vi "PerformanceAnalizer.vi"() -> ()   [LabVIEW 2010]
uses:
  <vilib>/picture/picture.llb/Draw True-Color Pixmap.vi
  <vilib>/Utility/file.llb/Write To Spreadsheet File (DBL).vi
  <vilib>/Utility/file.llb/Write To Spreadsheet File (string).vi
panel:
  out "KTH  Automatic Control \nCommunication performance analyzer":picture
  in  "Tab Control":T1(tab)
  out "reliability =pckSuccess/pckTotal":dynamicdata(graph)
  out "errors":dynamicdata(graph)
  out "Inter sampling time = t_k - t_k-1":dynamicdata(graph)
  out "delay = t_send - t_ack":dynamicdata(graph)
  out "lqi":dynamicdata(graph)
  out "rssi":dynamicdata(graph)
  out "rssi_0":i8
  out "rssi_1":i8
  out "rssi_2":i8
  out "lqi_0":i8
  out "lqi_1":i8
  out "lqi_2":i8
  in  "StartSaving":bool
  in  "Saving":bool
  in  "StopSaving":bool
  out "Path":path
  out "errors_0":dbl
  out "errors_2":dbl
  out "delay_1":dbl
  out "delay_0":dbl
  out "delay_2":dbl
  out "interSampling_1":dbl
  out "interSampling_3":dbl
  out "interSampling_0":dbl
  out "errors_1":dbl
  out "reliability_0":dbl
  out "reliability_1":dbl
  out "reliability_2":dbl
  out "current time":timestamp
  out "Packet Window":i32=200
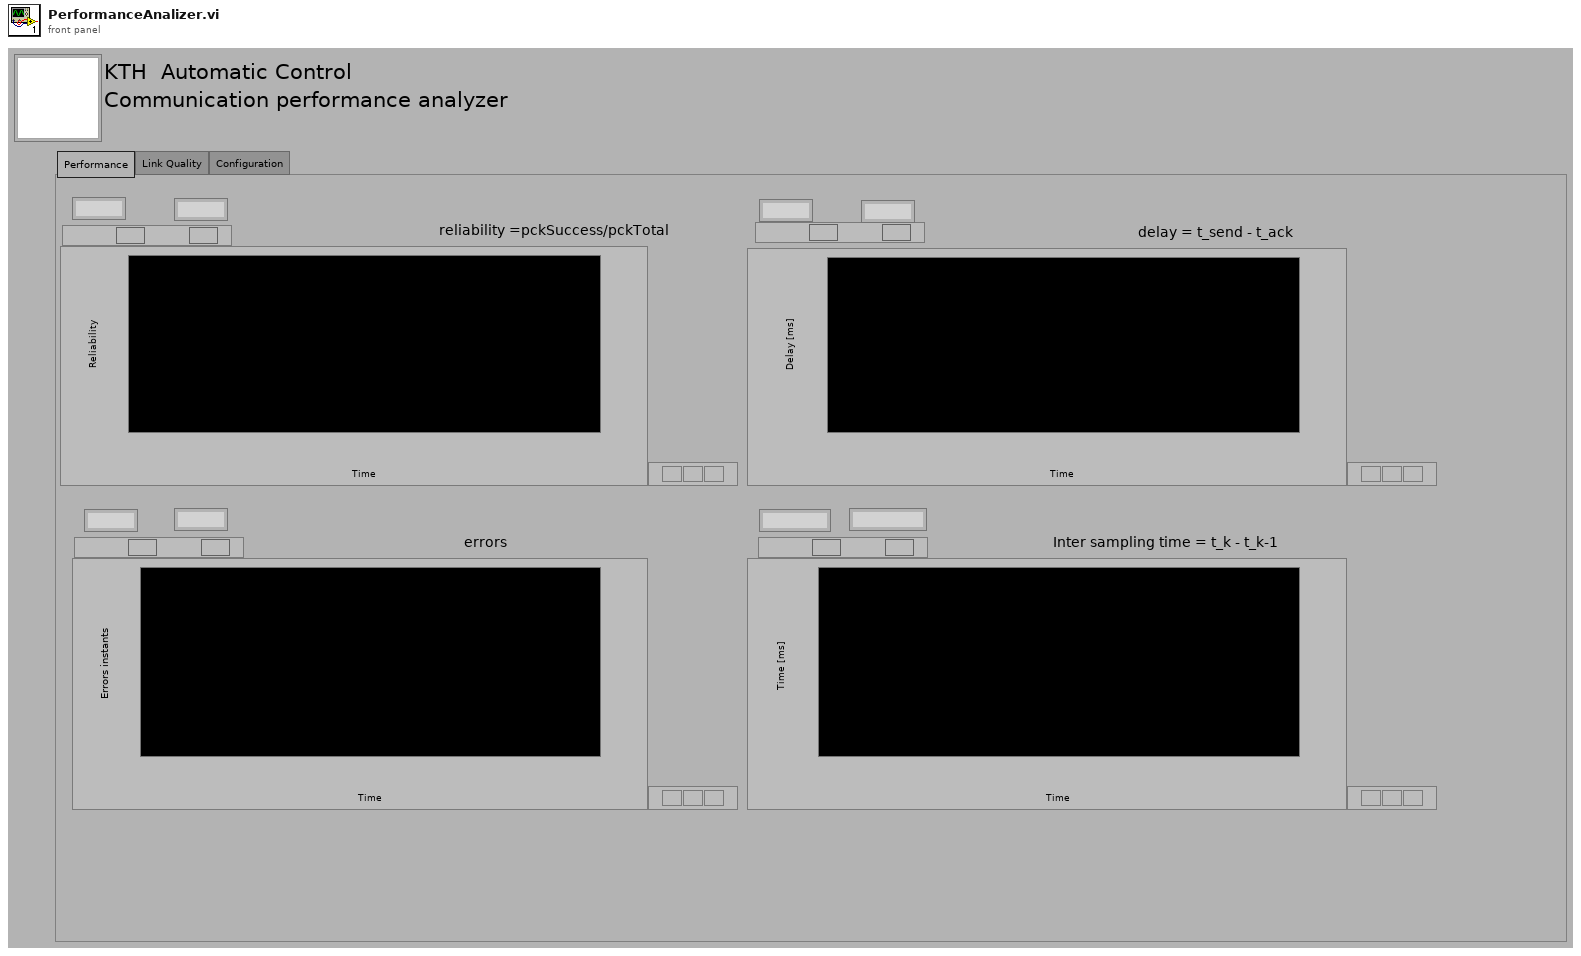
[diagram p1: front panel]
types:
  T1 = enum32{"Performance", "Link Quality", "Configuration"}
  T2 = enum8{"Enabled", "Disabled", "Disabled and Grayed Out"}
  T3 = typedef "imagedata.ctl" = cluster{"image type":i32, "image depth":i32, "image":u8[], "mask":u8[], "colors":u32[], "Rectangle":cluster{"left":i16, "top":i16, "right":i16, "bottom":i16}}
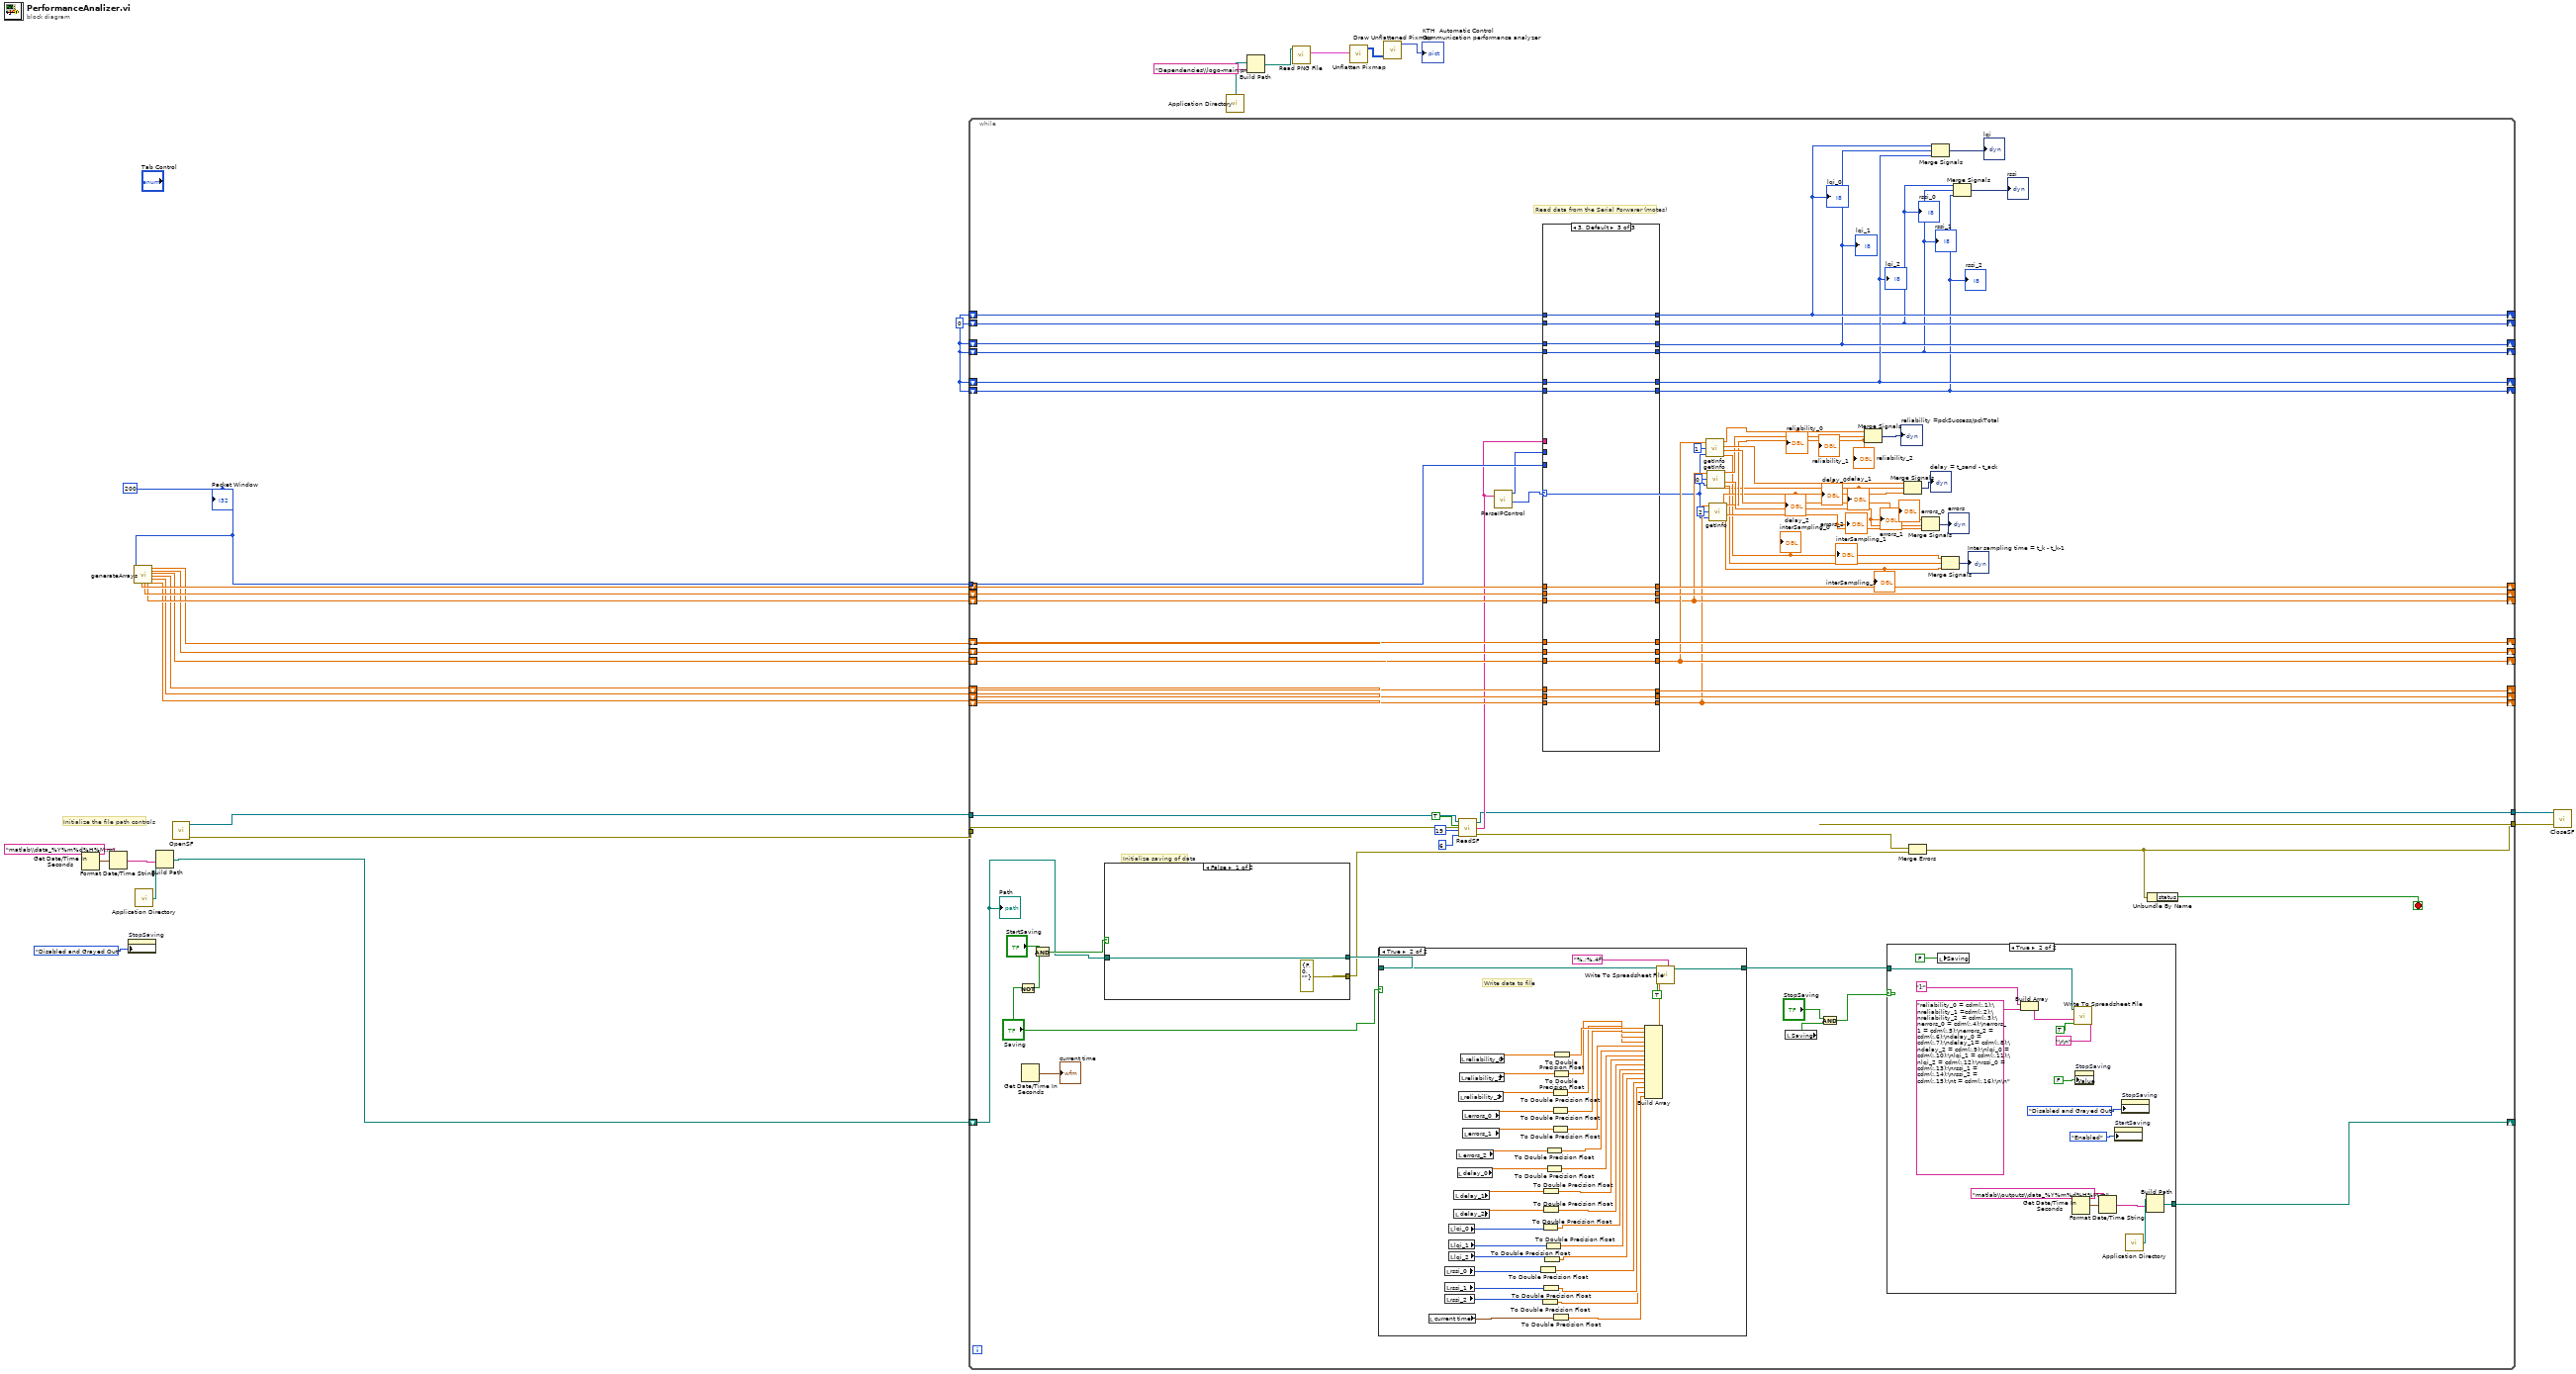
[diagram p0: block diagram]
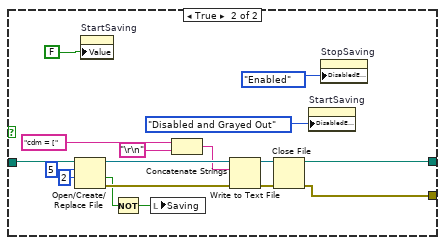
[diagram p4: hidden frame]
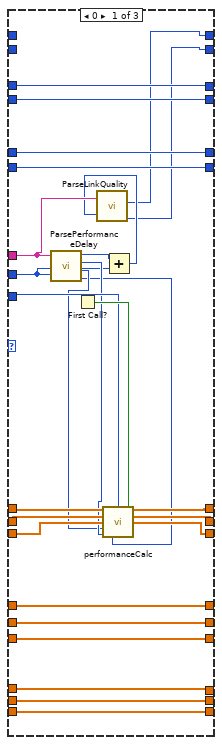
[diagram p5: hidden frame]
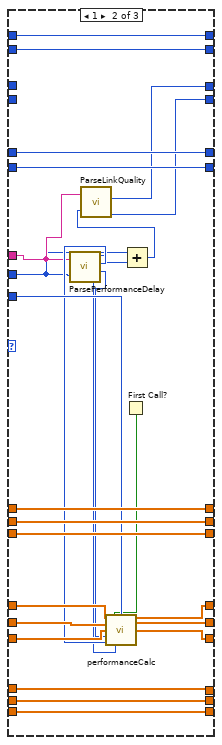
[diagram p6: hidden frame]
diagram:
  w1 = i8 0 ("rssi")
  w25 = 200 ("Packet Window")
  # "Initialize the file path controls"
  n1 = Get Date/Time In Seconds() -> (seconds since 1Jan1904=w14:timestamp)
  n2 = Format Date/Time String(time format string (%c)="matlab\\data_%Y%m%d%H%M.m", seconds (now)=w14) -> (date/time string=w12:string)  [unwired: 1 in]
  n3 = property on="StopSaving" class="Bool (strict)"("DisabledEnum"=T2."Disabled and Grayed Out" ("Disabled")) -> ()  [unwired: 2 in, 2 out]
  n4 = call "generateArrays.vi"("dimension size"=w25) -> ("errorsWindow1"=w24:dbl[], "pckTotalTrack1"=w23:dbl[], "state1"=w22:dbl[], "errorsWindow2"=w21:dbl[], "pckTotalTrack2"=w20:dbl[], "state2"=w19:dbl[], "errorsWindow3"=w18:dbl[], "pckTotalTrack3"=w17:dbl[], "state3"=w16:dbl[])  [unwired: 10 in]
  n5 = call <vilib>:"Application Directory.vi"() -> ("Application Directory"=w15:path)
  n6 = Build Path(base path=w15, name or relative path=w12) -> (appended path=w9:path)
  n7 = call "OpenSF.vi"() -> ("error out"=w26:errorcluster, "connection ID"=w27:refnum<k5>)  [unwired: 1 out]
  n8 = while {
    tunnel: w27 -> [w97]
    tunnel: w26 -> [w104]
    tunnel: [w60] -> w11
    tunnel: w25 -> [w100]
    shift-right: [w95] -> _
    shift-left: w24 -> [w93]
    shift-right: [w94] -> _
    shift-left: w23 -> [w92]
    shift-right: [w30] -> _
    shift-left: w22 -> [w91]
    shift-right: [w87] -> _
    shift-left: w21 -> [w90]
    shift-right: [w86] -> _
    shift-left: w20 -> [w89]
    shift-right: [w31] -> _
    shift-left: w19 -> [w88]
    shift-right: [w82] -> _
    shift-left: w18 -> [w85]
    shift-right: [w73] -> _
    shift-left: w17 -> [w84]
    shift-right: [w29] -> _
    shift-left: w16 -> [w83]
    shift-right: [w51] -> _
    shift-left: w9 -> [w50]
    tunnel: [w47] -> w2
    shift-right: [w32] -> _
    shift-left: w1 -> [w43]
    shift-right: [w35] -> _
    shift-left: w1 -> [w42]
    shift-right: [w36] -> _
    shift-left: w1 -> [w40]
    shift-right: [w33] -> _
    shift-left: w1 -> [w41]
    shift-right: [w37] -> _
    shift-left: w1 -> [w38]
    shift-right: [w34] -> _
    shift-left: w1 -> [w39]
    stop <- w59 stop-if-true
    # "Initialize saving of data"
    # "Read data from the Serial Forwarer (motes)"
    n9 = Not(x="Saving") -> (.not. x?=w56:bool)
    n10 = Get Date/Time In Seconds() -> (seconds since 1Jan1904=→"current time":timestamp)
    n11 = And(x="StartSaving", y=w56) -> (x .and. y?=w57:bool)
    n12 = case shown="False" w57 {
      tunnel: w50 -> [w160 w169]
      tunnel: [w160 w166] -> w65
      tunnel: [errorcluster {"status"=FALSE, "code"=0, "source"=""} ("error out") w163] -> w61
      frame False {
      }
      frame True {
        n13 = Open/Create/Replace File(file path (use dialog)=w169, operation (0:open)=5, access (0:read/write)=2) -> (refnum out=w175:refnum<file>, cancelled=w168:bool, error out=w172:errorcluster)  [unwired: 3 in]
        n14 = property on="StartSaving" class="Bool (strict)"("Value"=FALSE ("StartSaving")) -> ()  [unwired: 2 in, 2 out]
        n15 = Not(x=w168) -> (.not. x?=w165:bool)
        n16 = local write "Saving"(w165) -> ()
        n17 = Concatenate Strings("cdm = [", "\r\n") -> (w171:string)
        n18 = Write to Text File(file (use dialog)=w175, text=w171, error in=w172) -> (refnum out=w174:refnum<file>, error out=w173:errorcluster)  [unwired: 1 in, 1 out]
        n19 = Close File(refnum=w174, error in=w173) -> (path=w166:path, error out=w163:errorcluster)
        n20 = property on="StartSaving" class="Bool (strict)"("DisabledEnum"=T2."Disabled and Grayed Out" ("Disabled")) -> ()  [unwired: 2 in, 2 out]
        n21 = property on="StopSaving" class="Bool (strict)"("DisabledEnum"=T2."Enabled" ("Disabled")) -> ()  [unwired: 2 in, 2 out]
      }
    }
    n22 = case shown="True" "Saving" {
      tunnel: w65 -> [w121 w157]
      tunnel: [w121 w135] -> w62
      frame False {
      }
      frame True {
        # "Write data to file"
        n23 = local read "current time"() -> (w136:timestamp)
        n24 = local read "rssi_0"() -> (w128:i8)
        n25 = local read "rssi_1"() -> (w127:i8)
        n26 = local read "rssi_2"() -> (w126:i8)
        n27 = local read "lqi_0"() -> (w134:i8)
        n28 = local read "lqi_1"() -> (w133:i8)
        n29 = local read "lqi_2"() -> (w132:i8)
        n30 = local read "delay_1"() -> (w142:dbl)
        n31 = local read "delay_2"() -> (w143:dbl)
        n32 = local read "errors_2"() -> (w144:dbl)
        n33 = local read "delay_0"() -> (w145:dbl)
        n34 = local read "reliability_2"() -> (w152:dbl)
        n35 = local read "reliability_1"() -> (w153:dbl)
        n36 = local read "reliability_0"() -> (w155:dbl)
        n37 = local read "errors_0"() -> (w151:dbl)
        n38 = local read "errors_1"() -> (w148:dbl)
        n39 = To Double Precision Float(number=w128) -> (double precision float=w125:dbl)
        n40 = To Double Precision Float(number=w126) -> (double precision float=w123:dbl)
        n41 = To Double Precision Float(number=w134) -> (double precision float=w131:dbl)
        n42 = To Double Precision Float(number=w142) -> (double precision float=w139:dbl)
        n43 = To Double Precision Float(number=w143) -> (double precision float=w138:dbl)
        n44 = To Double Precision Float(number=w127) -> (double precision float=w124:dbl)
        n45 = To Double Precision Float(number=w132) -> (double precision float=w129:dbl)
        n46 = To Double Precision Float(number=w133) -> (double precision float=w130:dbl)
        n47 = To Double Precision Float(number=w144) -> (double precision float=w141:dbl)
        n48 = To Double Precision Float(number=w145) -> (double precision float=w140:dbl)
        n49 = To Double Precision Float(number=w152) -> (double precision float=w149:dbl)
        n50 = To Double Precision Float(number=w151) -> (double precision float=w147:dbl)
        n51 = To Double Precision Float(number=w148) -> (double precision float=w146:dbl)
        n52 = To Double Precision Float(number=w136) -> (double precision float=w122:dbl)
        n53 = To Double Precision Float(number=w153) -> (double precision float=w150:dbl)
        n54 = To Double Precision Float(number=w155) -> (double precision float=w154:dbl)
        n55 = Build Array(w154, w150, w149, w147, w146, w141, w140, w139, w138, w131, w130, w129, w125, w124, w123, w122) -> (w137:dbl[])
        n56 = call-poly <vilib>:"Write To Spreadsheet File.vi"("format (%.3f)"="%.;%.4f", "append to file? (new file:F)"=TRUE, "1D data"=w137, "file path (dialog if empty)"=w157) -> ("new file path (Not A Path if cancelled)"=w135:path)  [unwired: 4 in]
      }
    }
    n57 = call "ReadSF.vi"("connection ID in"=w97, "enabled"=TRUE, "bytes to read"=19 ("f"), "header size"=6 ("bytes to read"), "error in"=w104) -> ("connection ID out"=w47:refnum<k5>, "string"=w49:string, "error out"=w48:errorcluster)
    n58 = call "ParseIPControl.vi"("data out"=w49) -> ("srcId"=w28:u16, "Bytes Read"=w46:i32)  [unwired: 1 in, 2 out]
    n59 = case shown="3, Default" w28 {
      tunnel: w100 -> [w203 w222 _]
      tunnel: [w199 w231 w246] -> w95
      tunnel: [w198 w230 w245] -> w94
      tunnel: [w197 w229 w244] -> w30
      tunnel: w93 -> [w202 w231 w246]
      tunnel: w92 -> [w201 w230 w245]
      tunnel: w91 -> [w200 w229 w244]
      tunnel: w90 -> [w196 w225 w243]
      tunnel: w89 -> [w195 w224 w242]
      tunnel: w88 -> [w194 w223 w241]
      tunnel: [w196 w221 w243] -> w87
      tunnel: [w195 w220 w242] -> w86
      tunnel: [w194 w219 w241] -> w31
      tunnel: w85 -> [w193 w228 w240]
      tunnel: w84 -> [w192 w227 w239]
      tunnel: w83 -> [w191 w226 w238]
      tunnel: [w193 w228 w240] -> w82
      tunnel: [w192 w227 w239] -> w73
      tunnel: [w191 w226 w238] -> w29
      tunnel: w49 -> [w187 w214 _]
      tunnel: w46 -> [w186 w212 _]
      tunnel: [w183 w211 w232] -> w32
      tunnel: w43 -> [w183 w211 w232]
      tunnel: [w182 w210 w233] -> w35
      tunnel: [w181 w206 w234] -> w33
      tunnel: [w180 w207 w235] -> w36
      tunnel: [w178 w208 w236] -> w34
      tunnel: [w179 w209 w237] -> w37
      tunnel: w42 -> [w182 w210 w233]
      tunnel: w41 -> [w181 _ w234]
      tunnel: w40 -> [w180 _ w235]
      tunnel: w39 -> [_ w208 w236]
      tunnel: w38 -> [_ w209 w237]
      frame 0 {
        n60 = call "ParsePerformanceDelay.vi"("offset"=w186, "data out"=w187) -> ("delay"=w188:u16, "pckSuccess"=w189:u16, "pckTotal"=w190:u16, "Bytes Read"=w185:i32)
        n61 = First Call?() -> (First Call?: T/F=w204:bool)
        n62 = call "performanceCalc.vi"("errors"=w202, "init"=w204, "windowLength"=w203, "pckTotalTrack"=w201, "state"=w200, "pckSuccess"=w189, "pckTotal"=w190, "delay"=w188) -> ("errorsOut"=w199:dbl[], "pckTotalTrackOut"=w198:dbl[], "prevState"=w197:dbl[])  [unwired: 5 in]
        n63 = Add(x=w185, y=w186) -> (x+y=w184:i32)
        n64 = call "ParseLinkQuality.vi"("offset"=w184, "data out"=w187) -> ("rssi"=w178:i8, "LQI"=w179:i8)  [unwired: 2 out]
      }
      frame 1 {
        n65 = call "ParsePerformanceDelay.vi"("offset"=w212, "data out"=w214) -> ("delay"=w216:u16, "pckSuccess"=w215:u16, "pckTotal"=w217:u16, "Bytes Read"=w213:i32)
        n66 = First Call?() -> (First Call?: T/F=w218:bool)
        n67 = call "performanceCalc.vi"("errors"=w225, "init"=w218, "windowLength"=w222, "pckTotalTrack"=w224, "state"=w223, "pckSuccess"=w215, "pckTotal"=w217, "delay"=w216) -> ("errorsOut"=w221:dbl[], "pckTotalTrackOut"=w220:dbl[], "prevState"=w219:dbl[])  [unwired: 5 in]
        n68 = Add(x=w212, y=w213) -> (x+y=w205:i32)
        n69 = call "ParseLinkQuality.vi"("offset"=w205, "data out"=w214) -> ("rssi"=w206:i8, "LQI"=w207:i8)  [unwired: 2 out]
      }
      frame 3, Default {
      }
    }
    "lqi_2" <- w35
    "lqi_1" <- w36
    "lqi_0" <- w37
    "rssi_2" <- w32
    "rssi_1" <- w33
    "rssi_0" <- w34
    n70 = call "getInfo.vi"("array"=w31, "srcID"=u16 1, "srcIDPck"=w28) -> ("reliability"=w81:dbl, "delay"=w80:dbl, "errors"=w79:dbl, "interSampling"=w68:dbl)
    "reliability_0" <- w81
    "errors_0" <- w79
    "interSampling_0" <- w68
    "delay_0" <- w80
    n71 = call "getInfo.vi"("array"=w30, "srcID"=u16 0, "srcIDPck"=w28) -> ("reliability"=w78:dbl, "delay"=w64:dbl, "errors"=w77:dbl, "interSampling"=w67:dbl)
    "reliability_1" <- w78
    "errors_1" <- w77
    "interSampling_1" <- w67
    "delay_1" <- w64
    n72 = call "getInfo.vi"("array"=w29, "srcID"=u16 2, "srcIDPck"=w28) -> ("reliability"=w76:dbl, "delay"=w75:dbl, "errors"=w74:dbl, "interSampling"=w66:dbl)
    "reliability_2" <- w76
    "errors_2" <- w74
    "interSampling_3" <- w66
    "delay_2" <- w75
    n73 = local read "Saving"() -> (w52:bool)
    n74 = And(x="StopSaving", y=w52) -> (x .and. y?=w53:bool)
    n75 = Merge Signals(w81, w78, w76) -> (→"reliability =pckSuccess/pckTotal":dynamicdata)
    n76 = case shown="True" w53 {
      tunnel: w62 -> [w105 w113]
      tunnel: [w105 w106] -> w51
      frame False {
      }
      frame True {
        n77 = local write "Saving"(FALSE) -> ()
        n78 = Build Array("];", "reliability_0 = cdm(:,1);\nreliability_1 =cdm(:,2);\nreliability_2  = cdm(:,3);\nerrors_0 = cdm(:,4);\nerrors_1 = cdm(:,5);\nerrors_2 = cdm(:,6);\ndelay_0 = cdm(:,7);\ndelay_1= cdm(:,8);\ndelay_2 = cdm(:,9);\nlqi_0 = cdm(:,10);\nlqi_1 = cdm(:,11);\nlqi_2 = cdm(:,12);\nrssi_0 = cdm(:,13);\nrssi_1 = cdm(:,14);\nrssi_2 = cdm(:,15);\nt = cdm(:,16);\n\n") -> (w118:string[])
        n79 = Get Date/Time In Seconds() -> (seconds since 1Jan1904=w109:timestamp)
        n80 = call-poly <vilib>:"Write To Spreadsheet File.vi"("delimiter (\\t)"="\r\n", "append to file? (new file:F)"=TRUE, "1D data"=w118, "file path (dialog if empty)"=w113) -> ()  [unwired: 4 in, 1 out]
        n81 = property on="StopSaving" class="Bool (strict)"("Value"=FALSE ("StartSaving")) -> ()  [unwired: 2 in, 2 out]
        n82 = Format Date/Time String(time format string (%c)="matlab\\outputs\\data_%Y%m%d%H%M.m", seconds (now)=w109) -> (date/time string=w107:string)  [unwired: 1 in]
        n83 = property on="StartSaving" class="Bool (strict)"("DisabledEnum"=T2."Enabled" ("Disabled")) -> ()  [unwired: 2 in, 2 out]
        n84 = property on="StopSaving" class="Bool (strict)"("DisabledEnum"=T2."Disabled and Grayed Out" ("Disabled")) -> ()  [unwired: 2 in, 2 out]
        n85 = call <vilib>:"Application Directory.vi"() -> ("Application Directory"=w110:path)
        n86 = Build Path(base path=w110, name or relative path=w107) -> (appended path=w106:path)
      }
    }
    n87 = Merge Signals(w80, w64, w75) -> (→"delay = t_send - t_ack":dynamicdata)
    n88 = Merge Errors(w48, w61) -> (w60:errorcluster)
    n89 = Merge Signals(w79, w77, w74) -> (→"errors":dynamicdata)
    n90 = Merge Signals(w37, w36, w35) -> (→"lqi":dynamicdata)
    n91 = Merge Signals(w68, w67, w66) -> (→"Inter sampling time = t_k - t_k-1":dynamicdata)
    n92 = Merge Signals(w34, w33, w32) -> (→"rssi":dynamicdata)
    n93 = Unbundle By Name(w60) -> ("status"=w59:bool)
    "Path" <- w50
  }
  n94 = call <vilib>:"Application Directory.vi"() -> ("Application Directory"=w4:path)
  n95 = Build Path(base path=w4, name or relative path="Dependencies\\logo-main.png") -> (appended path=w5:path)
  n96 = call <vilib>:"Read PNG File.vi"("path to PNG file"=w5) -> ("image data"=w8:T3)  [unwired: 8 in, 2 out]
  n97 = call <vilib>:"Unflatten Pixmap.vi"("image data"=w8) -> ("24-bit pixmap"=w7:u32[][])  [unwired: 4 in, 6 out]
  n98 = call-poly <vilib>:"Draw Unflattened Pixmap.vi"("data (RGB format)"=w7) -> ("new picture"=→"KTH  Automatic Control \nCommunication performance analyzer":picture)  [unwired: 8 in]
  n99 = call "CloseSF.vi"("error out"=w11, "connection ID"=w2) -> ()  [unwired: 1 in]
  "Packet Window" <- w25
